vi "NI conSamp.vi"(2 "error in":errorcluster, 4 "Digitizer Settings":T1={"Digitizer delay (us) "=0.0, "rf points per line"=2048, "lines per plane"=128, "Samp Rate (Hz)"=100000000.0, "Additional dig delay (us)"=0.0, "Voltage Scale"=0.4, "Pre-Looks"=0, "Offset delay (us)"=0.0, "bits A/D"=8, "Avg Num"=1, "DigTimeOut"=5.0, "Rel Dig Delay"=0.0, "Dig Ch"=0, "LeCroyCluster"={"LeCroy Channels"=[TRUE, FALSE, FALSE, FALSE], "LC read pt offset"=0.0, "Sweep Avg"=FALSE}, "Main Digitizer"=enum."NI Digitizer", "Dig Config"=enum."Single channel", "Digitizer ID Cluster"={"Acqiris/Alazar/SP ID"=[], "NI Instr Handles"=[], "LeCroy VISA"="", "GaGe Handle"={"Handle"=0, "Sample size"=0, "Resolution"=0, "Offset"=0, "Channels"=0, "Boards"=0}, "ATS Ref"="ATS9350", "Acqiris Address"=["PCI::INSTR0"], "ADQRef"=refnum, "adq_cu_ptr"=refnum}, "Trigger Settings"={"Trig Source"=1, "Trig Coupling"=0, "Trig Slope"=0, "Level (mV)"=1500.0}, "Bulk Acq"=FALSE, "Bulk Start Indexes"=[], "Data Ref RF"=refnum, "NI ID/Channel"=[], "Total Dig CH"=1, "Xtra Ann Trig delay (us)"=10.0, "Fix Z Delay?"=FALSE, "One Way Transmission?"=FALSE, "Data Ref Log"=refnum} {"Trigger Settings"."Trig Slope" items=["Positive", "Negative"]; "Trigger Settings"."Level (mV)" format="%.2f"; "Trigger Settings"."Trig Coupling" items=["DC 1 MOhm", "AC 1 MOhm", "DC 50 Ohm", "AC 50 Ohm"]; "Trigger Settings"."Trig Source" items=["Chan 1", "External"]; "Rel Dig Delay" format="%.2f"; "DigTimeOut" format="%.2f"; "Avg Num" min=1; "Offset delay (us)" format="%.2f"; "Additional dig delay (us)" format="%.2f"; "Digitizer delay (us)" format="%.2f"}, 5 "InstrumentID":refnum<k15>) -> (0 "error out":errorcluster, 1 "DUP ID":refnum<k15>)   [LabVIEW 2022 SP3]
uses:
  -DigitizerRoutines/DigitizerSettings.ctl
  -DigitizerRoutines/Digitizer.ctl
  -DigitizerRoutines/DigConfig.ctl
  -DigitizerRoutines/DigitizerID.ctl
  C:/Windows/System32/ADQAPI_dotNet_helper.dll
panel:
  out "Acquisition:Binary Sample Width":i32
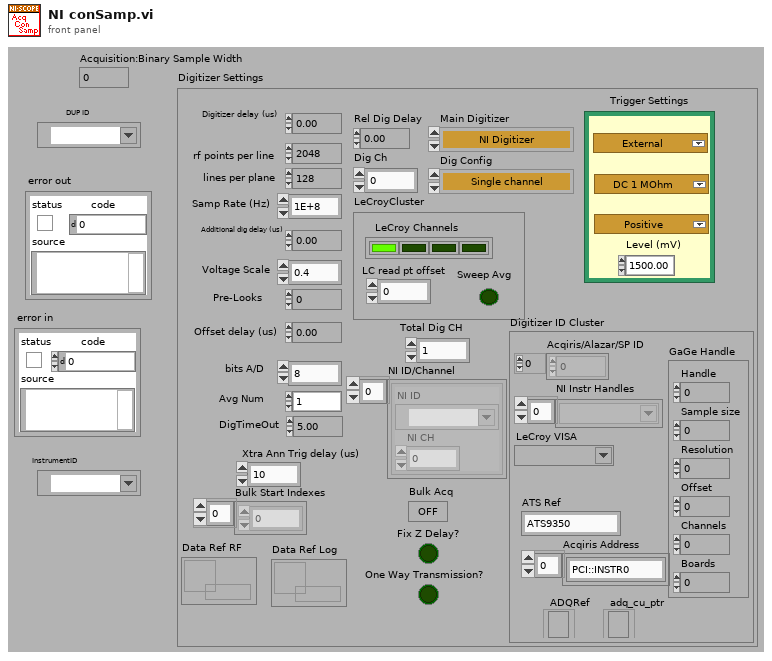
[diagram p1: front panel]
types:
  T1 = typedef "DigitizerSettings.ctl" = cluster{"Digitizer delay (us) ":dbl, "rf points per line":i32, "lines per plane":i32, "Samp Rate (Hz)":dbl, "Additional dig delay (us)":dbl, "Voltage Scale":dbl, "Pre-Looks":i32, "Offset delay (us)":dbl, "bits A/D":i8, "Avg Num":i32, "DigTimeOut":sgl, "Rel Dig Delay":sgl, "Dig Ch":i32, "LeCroyCluster":cluster{"LeCroy Channels":bool[], "LC read pt offset":dbl, "Sweep Avg":bool}, "Main Digitizer":T2, "Dig Config":T3, "Digitizer ID Cluster":T4, "Trigger Settings":cluster{"Trig Source":u16, "Trig Coupling":u16, "Trig Slope":u16, "Level (mV)":dbl}, "Bulk Acq":bool, "Bulk Start Indexes":i32[], "Data Ref RF":refnum<data-value>, "NI ID/Channel":cluster{"NI ID":refnum<k15>, "NI CH":i32}[], "Total Dig CH":i32, "Xtra Ann Trig delay (us)":dbl, "Fix Z Delay?":bool, "One Way Transmission?":bool, "Data Ref Log":refnum<data-value>}
  T2 = typedef "Digitizer.ctl" = enum16{"Acqiris Digitizer", "NI Digitizer", "LeCroy", "GaGe", "AlazarTech", "No Digitizer", "Teledyne"}
  T3 = typedef "DigConfig.ctl" = enum16{"Single channel", "2 Chans w/ 2 Acqiris", "2 Chans w/ 1 Acqiris", "5-CH Pulser New", "5-CH pulser w/ ann array", "5-pass style ann array", "Empty"}
  T4 = typedef "DigitizerID.ctl" = cluster{"Acqiris/Alazar/SP ID":u32[], "NI Instr Handles":refnum<k15>[], "LeCroy VISA":refnum<visa-resource-name>, "GaGe Handle":cluster{"Handle":u32, "Sample size":u32, "Resolution":i32, "Offset":i32, "Channels":u32, "Boards":u32}, "ATS Ref":string, "Acqiris Address":string[], "ADQRef":refnum<k24>, "adq_cu_ptr":refnum<k24>}
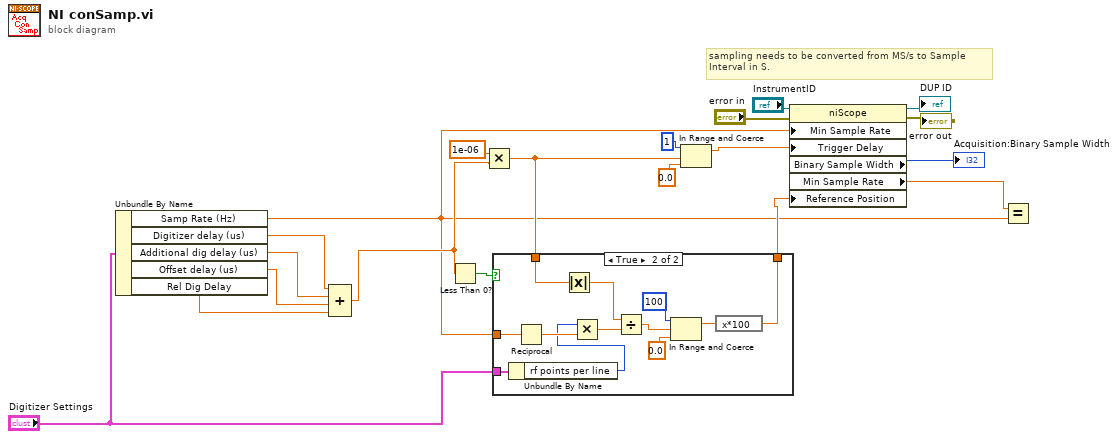
[diagram p0: block diagram]
diagram:
  # "sampling needs to be converted from MS/s to Sample\nInterval in S."
  n1 = Unbundle By Name("Digitizer Settings") -> ("Samp Rate (Hz)"=w2:dbl, "Digitizer delay (us)"=w7:dbl, "Additional dig delay (us)"=w6:dbl, "Offset delay (us)"=w5:dbl, "Rel Dig Delay"=w1:sgl)
  n2 = Compound Arithmetic op=ADD(w7, w6, w5, w1) -> (w3:dbl)
  n3 = Less Than 0?(x=w3) -> (x < 0?=w8:bool)
  n4 = Multiply(x=1e-06, y=w3) -> (x*y=w9:dbl)
  n5 = case shown="True" w8 {
    tunnel: w2 -> [_ w32]
    tunnel: w9 -> [_ w29]
    tunnel: [_ w23] -> w10
    tunnel: "Digitizer Settings" -> [_ w22]
    frame False {
    }
    frame True {
      n6 = Unbundle By Name(w22) -> ("rf points per line"=w21:i32)
      n7 = Reciprocal(x=w32) -> (1/x=w31:dbl)
      n8 = Absolute Value(x=w29) -> (abs(x)=w28:dbl)
      n9 = Multiply(x=w21, y=w31) -> (x*y=w30:dbl)
      n10 = Divide(x=w28, y=w30) -> (x/y=w26:dbl)
      n11 = In Range and Coerce(upper limit=100, x=w26, lower limit=0.0) -> (coerced(x)=w24:dbl)  [unwired: 1 out]
      n12 = expression code="x*100"(w24) -> (w23:dbl)
    }
  }
  n13 = In Range and Coerce(upper limit=1, x=w9, lower limit=0.0) -> (coerced(x)=w13:dbl)  [unwired: 1 out]
  n14 = property class="niScope"(reference="InstrumentID", error in="error in", "Min Sample Rate"=w2, "Trigger Delay"=w13, "Reference Position"=w10) -> (reference out=→"DUP ID":refnum<k15>, error out=→"error out":errorcluster, "Binary Sample Width"=→"Acquisition:Binary Sample Width":i32, "Min Sample Rate"=w14:dbl)
  n15 = Equal?(x=w14, y=w2) -> ()  [unwired: 1 out]
